vi "Latihan 6 (While Loop).vi"() -> ()   [LabVIEW 2021]
panel:
  out "Numeric 2":i32
  in  "stop":bool
  out "Numeric":dbl
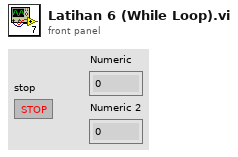
[diagram p1: front panel]
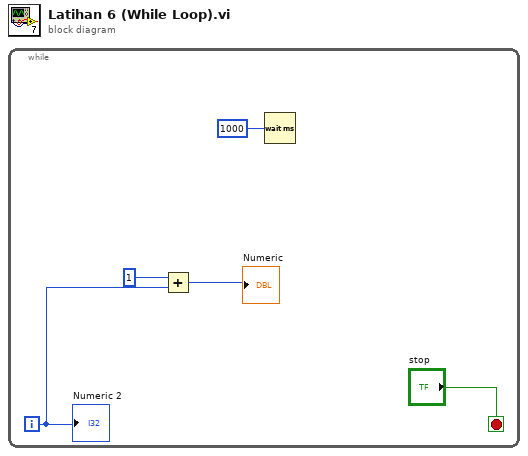
[diagram p0: block diagram]
diagram:
  n1 = while {
    i -> [w3]
    stop <- "stop" stop-if-true
    n2 = Add(x=1, y=w3) -> (x+y=→"Numeric":i32)
    n3 = Wait (ms)(milliseconds to wait=u32 1000) -> ()  [unwired: 1 out]
    "Numeric 2" <- w3
  }
